vi "Drive Toggle.vi"(10 "Limit":i32, 11 "Button":bool) -> (3 "Output":i32)   [LabVIEW 2014]
doc: "This vi. Takes the button value and counts it. Once count is greater then \"limit\" the count reset to 0."
uses:
  <vilib>/ptbypt/NI_PtbyPt.lvlib
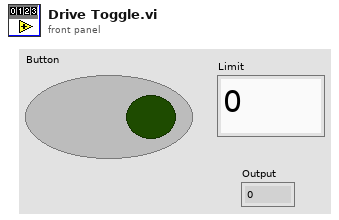
[diagram p1: front panel]
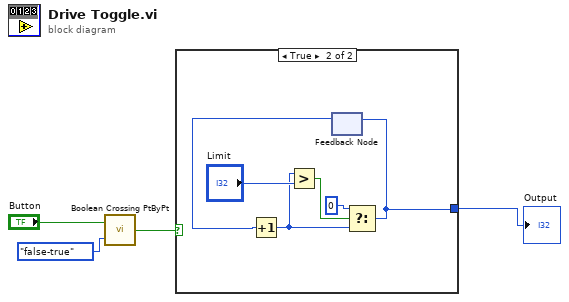
[diagram p0: block diagram]
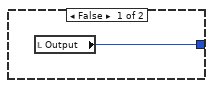
[diagram p2: hidden frame]
diagram:
  n1 = call <vilib>:"Boolean Crossing PtByPt.vi"("direction"=enum16{"either", "false-true", "true-false"}."false-true", "input"="Button") -> ("crossing"=w3:bool)  [unwired: 1 in]
  n2 = case shown="True" w3 {
    tunnel: [w5 w6] -> w1
    frame False {
      n3 = local read "Output"() -> (w5:i32)
    }
    frame True {
      n4 = feedback #1() -> (w11:i32)  [unwired: 1 in]
      n5 = Increment(x=w11) -> (x+1=w7:i32)
      n6 = Greater?(x=w7, y="Limit") -> (0:w9:bool)
      n7 = Select(t=0, s=w9, f=w7) -> (s? t:f=w6:i32)
      n8 = feedback-in #1(w6) -> ()
    }
  }
  "Output" <- w1
